vi "stage_move.vi"(0 "Sys_num":i32=1, 1 "Start":dbl=50.0, 2 "Stop":dbl=51.0, 3 "No.of digits":i16=4, 4 "Gap":dbl=0.5, 5 "Conn. Axes":string[](array[string]), 6 "Stop ref":refnum<vi>, 7 "stage_num":i32, 9 "position ref":refnum<vi>, 11 "Stage error in":errorcluster, 12 "Moving Velocity":dbl=1.5, 13 "Final Velocity":dbl=1.5, 14 "polling time":u32=100) -> (8 "Final position":dbl, 10 "Direction":bool, 15 "Stage error out":errorcluster)   [LabVIEW 2014]
doc: "This vi will move the stage to the desitination, AND the stage approachs the destination from defined direction depending the direction-flag. Step determines the overshoot distance.\nAfter this, the velocity is set to final velocity for further small step measurements."
uses:
  <vilib>/Utility/error.llb/DialogType.ctl
panel:
  out "Position":dbl[](array[numeric]) format="%.6f"
  in  "stop":bool
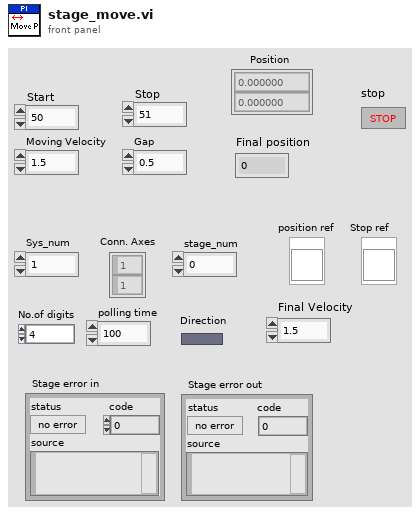
[diagram p1: front panel]
types:
  T1 = typedef "DialogType.ctl" = u16
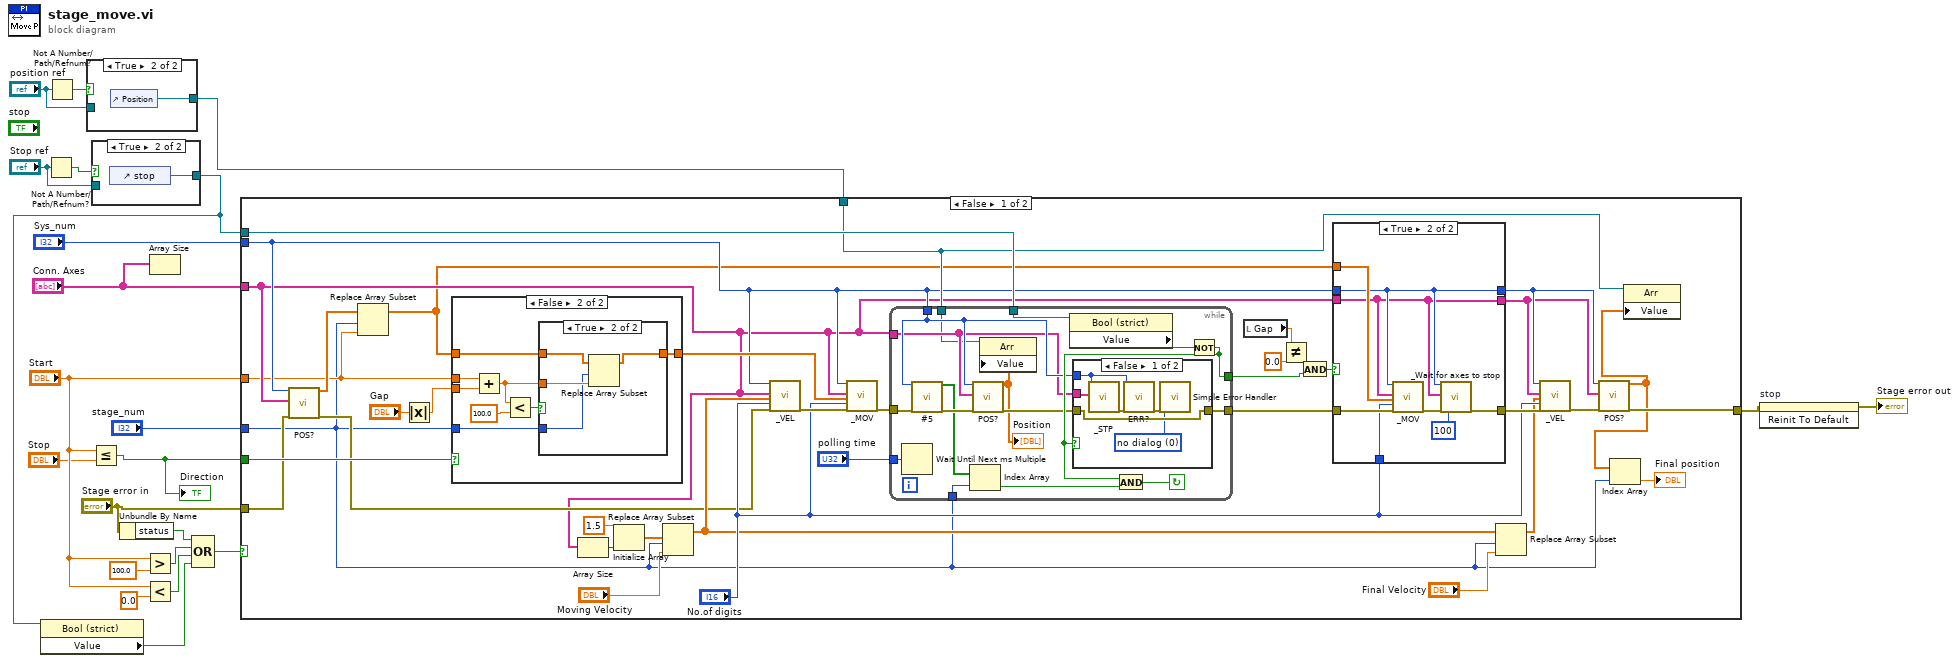
[diagram p0: block diagram]
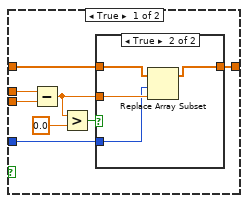
[diagram p6: hidden frame]
diagram:
  n1 = Not A Number/Path/Refnum?(number/path/refnum="Stop ref") -> (NaN/Path/Refnum?=w10:bool)
  n2 = Not A Number/Path/Refnum?(number/path/refnum="position ref") -> (NaN/Path/Refnum?=w6:bool)
  n3 = case shown="True" w6 {
    tunnel: [w23 w24] -> w1
    tunnel: "position ref" -> [w23 _]
    frame False {
    }
    frame True {
      n4 = control-ref of="Position"() -> (w24:refnum<vi>)
    }
  }
  n5 = Less Or Equal?(x="Start", y="Stop") -> (x <= y?=w11:bool)
  "Direction" <- w11
  n6 = case shown="True" w10 {
    tunnel: [w25 w26] -> w8
    tunnel: "Stop ref" -> [w25 _]
    frame False {
    }
    frame True {
      n7 = control-ref of="stop"() -> (w26:refnum<vi>)
    }
  }
  n8 = property class="Bool (strict)"(reference=w8) -> ("Value"=w7:bool)  [unwired: 1 in, 2 out]
  n9 = Unbundle By Name("Stage error in") -> ("status"=w20:bool)
  n10 = Greater?(x="Start", y=100.0) -> (0:w18:bool)
  n11 = Less?(x="Start", y=0.0) -> (x < y?=w17:bool)
  n12 = Array Size(array="Conn. Axes") -> ()  [unwired: 1 out]
  n13 = Compound Arithmetic op=OR(w20, w18, w17, w7) -> (w19:bool)
  n14 = case shown="False" w19 {
    tunnel: [w41 w125] -> w4
    tunnel: "stage_num" -> [w28 _]
    tunnel: "Start" -> [w29 _]
    tunnel: "Stage error in" -> [w34 w125]
    tunnel: "Conn. Axes" -> [w31 _]
    tunnel: w11 -> [w49 _]
    tunnel: w8 -> [w48 _]
    tunnel: w1 -> [w38 _]
    tunnel: "Sys_num" -> [w32 _]
    frame False {
      n15 = call "POS?.vi"("System no."=w32, "Axes to query"=w31, "error in"=w34) -> ("Position"=w30:dbl[], "error out"=w33:errorcluster)  [unwired: 15 in]
      n16 = Replace Array Subset(array=w30, new element=w29, index=w28) -> (w27:dbl[])
      n17 = Absolute Value(x="Gap") -> (abs(x)=w63:dbl)
      n18 = case shown="False" w49 {
        tunnel: w29 -> [w106 w119]
        tunnel: w28 -> [w102 w115]
        tunnel: w27 -> [w101 w114]
        tunnel: [w100 w113] -> w59
        tunnel: w63 -> [w99 w112]
        frame True {
          n19 = Subtract(x=w106, y=w99) -> (x-y=w103:dbl)
          n20 = Greater?(x=w103, y=0.0) -> (0:w105:bool)
          n21 = case shown="True" w105 {
            tunnel: w103 -> [_ w111]
            tunnel: w102 -> [_ w110]
            tunnel: w101 -> [w107 w109]
            tunnel: [w107 w108] -> w100
            frame False {
            }
            frame True {
              n22 = Replace Array Subset(array=w109, new element=w111, index=w110) -> (w108:dbl[])
            }
          }
        }
        frame False {
          n23 = Add(x=w119, y=w112) -> (x+y=w116:dbl)
          n24 = Less?(x=w116, y=100.0) -> (x < y?=w118:bool)
          n25 = case shown="True" w118 {
            tunnel: w116 -> [_ w124]
            tunnel: w115 -> [_ w123]
            tunnel: w114 -> [w120 w122]
            tunnel: [w120 w121] -> w113
            frame False {
            }
            frame True {
              n26 = Replace Array Subset(array=w122, new element=w124, index=w123) -> (w121:dbl[])
            }
          }
        }
      }
      n27 = Array Size(array=w31) -> (size(s)=w58:i32)
      n28 = Initialize Array(1.5 ("element"), w58) -> (w56:dbl[])
      n29 = Replace Array Subset(array=w56, new element="Moving Velocity", index=w28) -> (w52:dbl[])
      n30 = call "_VEL.vi"("System no."=w32, "Axes to set"=w31, "Velocity values"=w52, "No.of digits"="No.of digits", "error in"=w33) -> ("error out"=w62:errorcluster)  [unwired: 13 in, 1 out]
      n31 = call "_MOV.vi"("System no."=w32, "Axes to move"=w31, "Position values"=w59, "No.of digits"="No.of digits", "error in"=w62) -> ("error out"=w61:errorcluster)  [unwired: 14 in]
      n32 = while {
        tunnel: w61 -> [w83]
        tunnel: "polling time" -> [w91]
        tunnel: w32 -> [w79]
        tunnel: w31 -> [w78]
        tunnel: [w85] -> w35
        tunnel: w38 -> [w77]
        tunnel: w28 -> [w90]
        tunnel: w48 -> [w89]
        tunnel: [w84] -> w43
        stop <- w87 continue-if-true
        n33 = Wait Until Next ms Multiple(millisecond multiple=w91) -> ()  [unwired: 1 out]
        n34 = call "#5.vi"("System no."=w79, "error in"=w83) -> ("Axis moving?"=w80:bool[], "error out"=w82:errorcluster)  [unwired: 16 in]
        n35 = Index Array(array=w80, index=w90) -> (element=w88:bool)
        n36 = call "POS?.vi"("System no."=w79, "Axes to query"=w78, "error in"=w82) -> ("Position"=w76:dbl[], "error out"=w81:errorcluster)  [unwired: 15 in]
        "Position" <- w76
        n37 = property class="Arr"(reference=w77, "Value"=w76) -> ()  [unwired: 1 in, 2 out]
        n38 = property class="Bool (strict)"(reference=w89) -> ("Value"=w86:bool)  [unwired: 1 in, 2 out]
        n39 = Not(x=w86) -> (.not. x?=w84:bool)
        n40 = case shown="False" w84 {
          tunnel: [w94 w98] -> w85
          tunnel: w81 -> [w94 w98]
          tunnel: w79 -> [w95 _]
          tunnel: w78 -> [w97 _]
          frame False {
            w92 = T1 0 items=["no dialog", "OK message", "continue or stop message", "OK message + warnings", "continue/stop + warnings"] ("type of dialog (OK msg:1)")
            n41 = call "_STP.vi"("System no."=w95, "Affected axes?"=w97) -> ("error out"=w96:errorcluster)  [unwired: 17 in]
            n42 = call "ERR?.vi"("System no."=w95, "error in"=w96) -> ("error out"=w93:errorcluster)  [unwired: 16 in, 1 out]
            n43 = call <vilib>:"Simple Error Handler.vi"("type of dialog (OK msg:1)"=w92, "error in (no error)"=w93) -> ()  [unwired: 3 in, 5 out]
          }
          frame True {
          }
        }
        n44 = And(x=w84, y=w88) -> (x .and. y?=w87:bool)
      }
      n45 = local read "Gap"() -> (w47:dbl)
      n46 = Not Equal?(x=w47, y=0.0) -> (x != y?=w45:bool)
      n47 = And(x=w45, y=w43) -> (x .and. y?=w44:bool)
      n48 = case shown="True" w44 {
        tunnel: w35 -> [w67 w75]
        tunnel: w27 -> [_ w74]
        tunnel: [w67 w70] -> w54
        tunnel: "No.of digits" -> [_ w73]
        tunnel: w32 -> [w66 w69]
        tunnel: w31 -> [w65 w68]
        tunnel: [w66 w69] -> w37
        tunnel: [w65 w68] -> w36
        frame False {
        }
        frame True {
          n49 = call "_MOV.vi"("System no."=w69, "Axes to move"=w68, "Position values"=w74, "No.of digits"=w73, "error in"=w75) -> ("error out"=w72:errorcluster)  [unwired: 14 in]
          n50 = call "_Wait for axes to stop.vi"("System no."=w69, "Axes to wait for"=w68, "error in"=w72, "Polling cycle time, ms"=u32 100) -> ("error out"=w70:errorcluster)  [unwired: 14 in, 1 out]
        }
      }
      n51 = Replace Array Subset(array=w52, new element="Final Velocity", index=w28) -> (w50:dbl[])
      n52 = call "_VEL.vi"("System no."=w37, "Axes to set"=w36, "Velocity values"=w50, "No.of digits"="No.of digits", "error in"=w54) -> ("error out"=w42:errorcluster)  [unwired: 13 in, 1 out]
      n53 = call "POS?.vi"("System no."=w37, "Axes to query"=w36, "error in"=w42) -> ("Position"=w39:dbl[], "error out"=w41:errorcluster)  [unwired: 15 in]
      n54 = Index Array(array=w39, index=w28) -> (element=→"Final position":dbl)
      n55 = property class="Arr"(reference=w38, "Value"=w39) -> ()  [unwired: 1 in, 2 out]
    }
    frame True {
    }
  }
  n56 = invoke on="stop" class="Bool (strict)" method="Reinit To Default"(error in=w4) -> (error out=→"Stage error out":errorcluster)  [unwired: 2 in, 2 out]
